vi "Car Go Right.vi"(9 "m array":i16[][](array[numeric]), 10 "Numeric":i32, 11 "Input in":i32[][](array[numeric])) -> (2 "move or not":bool, 3 "Input out":i32[][](array[numeric]))   [LabVIEW 2021]
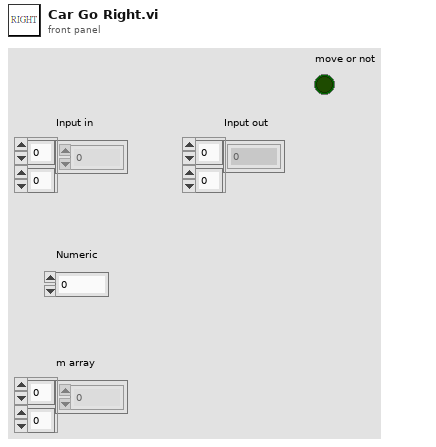
[diagram p1: front panel]
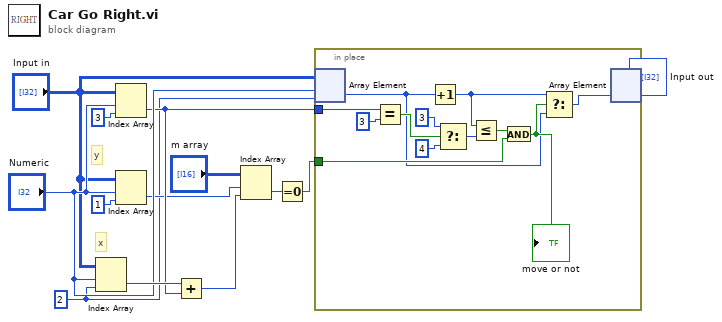
[diagram p0: block diagram]
diagram:
  w2 = 2
  # "x"
  # "y"
  n1 = Index Array(array="Input in", index (row)="Numeric", index (col)=w2) -> (element=w13:i32)
  n2 = Index Array(array="Input in", index (row)="Numeric", index (col)=3 ("disabled index (col)")) -> (element=w9:i32)
  n3 = Index Array(array="Input in", index (row)="Numeric", index (col)=1 ("disabled index (col)")) -> (element=w7:i32)
  n4 = Add(x=w13, y=w9) -> (x+y=w8:i32)
  n5 = Index Array(array="m array", index (row)=w7, index (col)=w8) -> (element=w1:i16)
  n6 = Equal To 0?(x=w1) -> (x = 0?=w10:bool)
  n7 = in-place {
    in-place-border: w9 -> [w23]
    in-place-border: w10 -> [w15]
    n8 = in-place-array #1("Input in", "Numeric", w2) -> (w14:i32)
    n9 = Equal?(x=w23, y=3) -> (x = y?=w21:bool)
    n10 = Increment(x=w14) -> (x+1=w24:i32)
    n11 = Select(t=3 ("y"), s=w21, f=4) -> (s? t:f=w18:i32)
    n12 = Less Or Equal?(x=w24, y=w18) -> (x <= y?=w16:bool)
    n13 = And(x=w16, y=w15) -> (x .and. y?=w17:bool)
    "move or not" <- w17
    n14 = Select(t=w24, s=w17, f=w14) -> (s? t:f=w25:i32)
    n15 = in-place-array #1(w25) -> (→"Input out":i32[][])  [unwired: 2 out]
  }
